vi "Show phase.vi"(6 "offset":dbl, 7 "Which phase":enum16{"Sine", "Stimulus"}(ring), 8 "start time":timestamp, 9 "stimphases":T1, 10 "motor":waveform(dbl), 11 "voltage":waveform(dbl)[](array[waveform])) -> (3 "plots":cluster{"Y":dbl[], dbl[]}[](array[cluster]))   [LabVIEW 2013]
uses:
  Stim phases.ctl
  <vilib>/Waveform/WDTOps.llb/WDT Waveform Duration DBL.vi
  <vilib>/Waveform/WDTOps.llb/WDT Get Waveform Subset DBL.vi
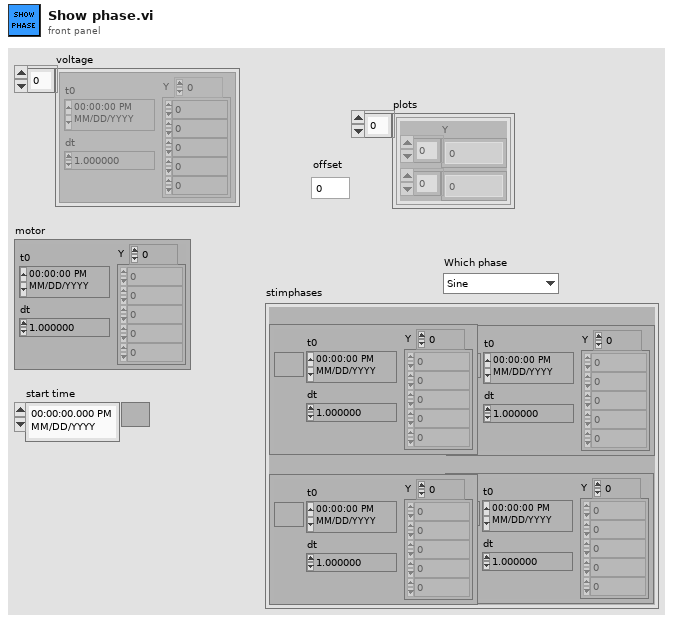
[diagram p1: front panel]
types:
  T1 = typedef "Stim phases.ctl" = cluster{"sinephase":waveform(dbl), "sinecycles":waveform(dbl), "stimphase":waveform(dbl), "stimcycles":waveform(dbl)}
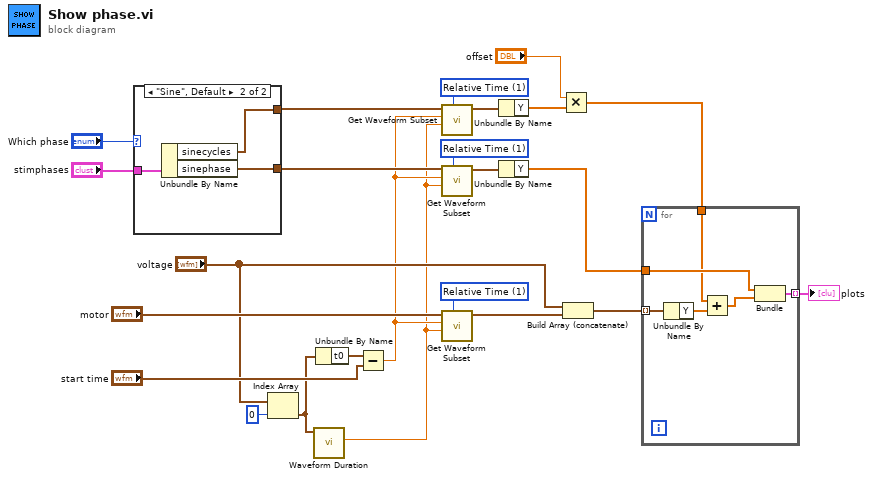
[diagram p0: block diagram]
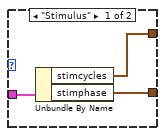
[diagram p2: hidden frame]
diagram:
  w8 = u16 1 items=["Samples", "Relative Time"] ("start/duration format")
  w16 = u16 1 items=["Samples", "Relative Time"] ("start/duration format")
  w22 = u16 1 items=["Samples", "Relative Time"] ("start/duration format")
  n1 = case shown="\"Sine\", Default" "Which phase" {
    tunnel: "stimphases" -> [w27 w30]
    tunnel: [w26 w29] -> w15
    tunnel: [w25 w28] -> w7
    frame "Stimulus" {
      n2 = Unbundle By Name(w27) -> ("stimcycles"=w25:waveform(dbl), "stimphase"=w26:waveform(dbl))
    }
    frame "Sine", Default {
      n3 = Unbundle By Name(w30) -> ("sinecycles"=w28:waveform(dbl), "sinephase"=w29:waveform(dbl))
    }
  }
  n4 = Index Array(array="voltage", index=0) -> (element=w20:waveform(dbl))
  n5 = call-poly <vilib>:"Waveform Duration.vi"("waveform in"=w20) -> ("duration"=w5:dbl)  [unwired: 8 in, 2 out]
  n6 = Unbundle By Name(w20) -> ("t0"=w23:timestamp)
  n7 = Subtract(x=w23, y="start time") -> (x-y=w6:dbl)
  n8 = call-poly <vilib>:"Get Waveform Subset.vi"("start/duration format"=w8, "duration"=w5, "start samples/time"=w6, "waveform in"=w7) -> ("waveform out"=w9:waveform(dbl))  [unwired: 2 in, 3 out]
  n9 = call-poly <vilib>:"Get Waveform Subset.vi"("start/duration format"=w16, "duration"=w5, "start samples/time"=w6, "waveform in"=w15) -> ("waveform out"=w14:waveform(dbl))  [unwired: 2 in, 3 out]
  n10 = call-poly <vilib>:"Get Waveform Subset.vi"("start/duration format"=w22, "duration"=w5, "start samples/time"=w6, "waveform in"="motor") -> ("waveform out"=w13:waveform(dbl))  [unwired: 2 in, 3 out]
  n11 = Unbundle By Name(w9) -> ("Y"=w4:dbl[])
  n12 = Unbundle By Name(w14) -> ("Y"=w10:dbl[])
  n13 = Multiply(x="offset", y=w4) -> (x*y=w2:dbl[])
  n14 = Build Array (concatenate)("voltage", w13) -> (w11:waveform(dbl)[])
  n15 = for {
    tunnel: w11 -> [w36] mode=indexing
    tunnel: w10 -> [w35]
    tunnel: [w34] -> w1 mode=indexing
    tunnel: w2 -> [w32]
    n16 = Unbundle By Name(w36) -> ("Y"=w33:dbl[])
    n17 = Add(x=w32, y=w33) -> (x+y=w31:dbl[])
    n18 = Bundle("Y"=w35, w31) -> (w34:cluster{"Y":dbl[], dbl[]})  [unwired: 1 in]
  }
  "plots" <- w1
